vi "Create AVI FName (SubVI).vi"(10 "Save":bool, 11 "Movie File Path":path) -> (2 "Image REF":T2, 3 "AVI Refnum":T1)   [LabVIEW 2020]
uses:
  <vilib>/vision/Image Controls.llb/IMAQ Image.ctl
  <vilib>/vision/Avi.llb/IMAQ AVI2 Refnum.ctl
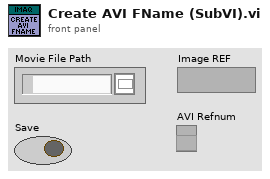
[diagram p1: front panel]
types:
  T1 = typedef "IMAQ AVI2 Refnum.ctl" = refnum<k20>
  T2 = typedef "IMAQ Image.ctl" = refnum<image>
  T3 = typedef "Image Type" = u32
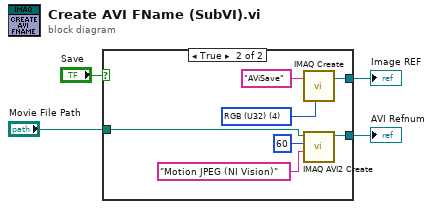
[diagram p0: block diagram]
diagram:
  n1 = case shown="True" "Save" {
    tunnel: [_ w11] -> w1
    tunnel: [_ w10] -> w2
    tunnel: "Movie File Path" -> [_ w7]
    frame False {
    }
    frame True {
      w5 = T3 4 items=["Grayscale (U8)", "Grayscale (I16)", "Grayscale (SGL)", "Complex (CSG)", "RGB (U32)", "HSL (U32)", "RGB (U64)", "Grayscale (U16)"] ("Image Type")
      n2 = call "IMAQ Create"("Image Name"="AViSave", "Image Type"=w5) -> ("New Image"=w10:T2)  [unwired: 3 in, 1 out]
      n3 = call "IMAQ AVI2 Create"("Codec"="Motion JPEG (NI Vision)" ("CODEC"), "Frames Per Second"=u32 60, "AVI Path"=w7) -> ("AVI Refnum"=w11:T1)  [unwired: 7 in, 1 out]
    }
  }
  "Image REF" <- w2
  "AVI Refnum" <- w1
